vi "Data Bingding.vi"(8 "error in (no error)":errorcluster caption="错误输入（无错误）", 10 "dataMember":string, 11 "DataSet 输入":refnum<class "DataSet.lvclass"> caption="DNL_LabVIEW Object in") -> (0 "error out":errorcluster caption="错误输出", 3 "DataSet 输出":refnum<class "DataSet.lvclass"> caption="DNL_LabVIEW Object out")   [LabVIEW 2012, in "Data Grid VIEW.lvlib" / "DataSet.lvclass"]
uses:
  DataSet.lvclass
  DataSet.lvclass/DataSet.ctl
  System.Windows.Forms
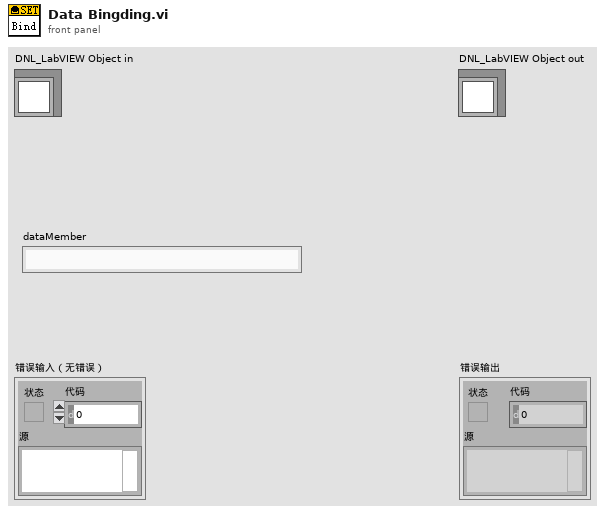
[diagram p1: front panel]
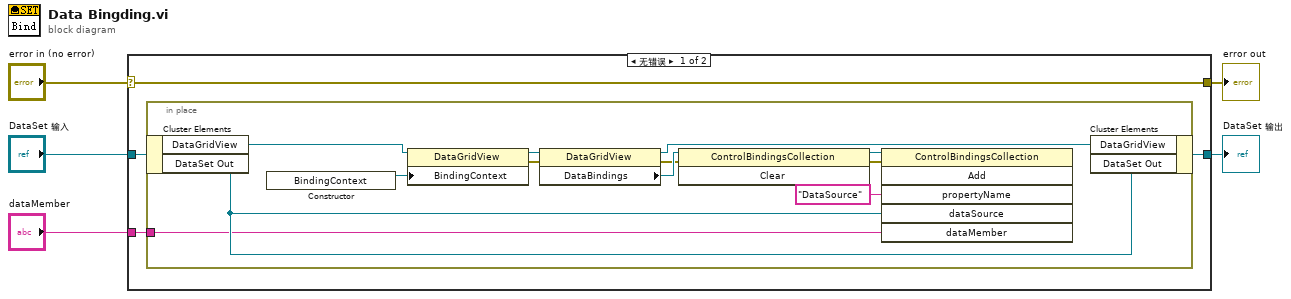
[diagram p0: block diagram]
diagram:
  n1 = case shown="无错误" "error in (no error)" {
    selector: "error in (no error)" -> [w9 w23]
    tunnel: [w9 w23] -> w4
    tunnel: "DataSet 输入" -> [w8 w22]
    tunnel: "dataMember" -> [w7 _]
    tunnel: [w6 w22] -> w1
    frame No Error {
      n2 = in-place {
        in-place-border: w7 -> [w15]
        n3 = in-place-cluster #1(w8) -> ("DataGridView"=w17:refnum<k24>, "DataSet Out"=w16:refnum<k24>)
        n4 = constructor class="BindingContext"() -> (reference out=w21:refnum<k24>)  [unwired: 3 in, 2 out]
        n5 = property class="DataGridView"(reference=w17, "BindingContext"=w21) -> (reference out=w18:refnum<k24>, error out=w19:errorcluster)  [unwired: 1 in]
        n6 = property class="DataGridView"(reference=w18, error in=w19) -> (reference out=w14:refnum<k24>, error out=w11:errorcluster, "DataBindings"=w13:refnum<k24>)
        n7 = invoke class="ControlBindingsCollection" method="Clear"(reference=w13, error in=w11) -> (reference out=w12:refnum<k24>, error out=w10:errorcluster)  [unwired: 1 in, 1 out]
        n8 = invoke class="ControlBindingsCollection" method="Add"(reference=w12, error in=w10, "propertyName"="DataSource", "dataSource"=w16, "dataMember"=w15) -> ()  [unwired: 1 in, 6 out]
        n9 = in-place-cluster #1("DataGridView"=w14, "DataSet Out"=w16) -> (w6:refnum<class "DataSet.lvclass">)
      }
    }
    frame Error {
    }
  }
  "error out" <- w4
  "DataSet 输出" <- w1
